vi "get.vi"(8 "variableArray":string[][](array[string]), 10 "variables":string[](array[string])=["intout", "stringout", "time"], 11 "Experience ID":string="Test") -> (0 "error out":errorcluster={"status"=TRUE, "code"=1, "source"="Entry not found"}, 2 "values":string[](array[string])=["0"], 3 "names":string[](array[string])=["intout"], 5 "values 2":string[](array[string])=["0"], 7 "names 2":string[](array[string])=["intout"])   [LabVIEW 2020]
panel:
  # "Get"
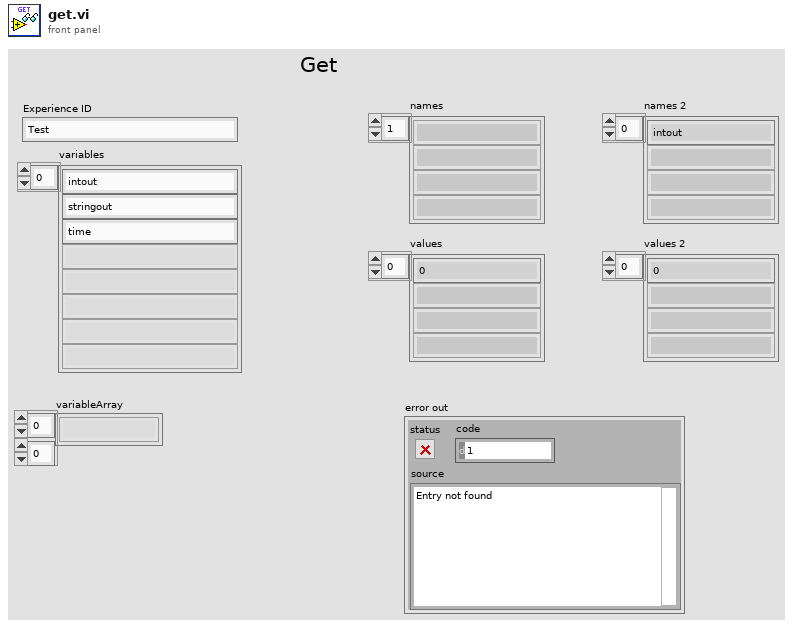
[diagram p1: front panel]
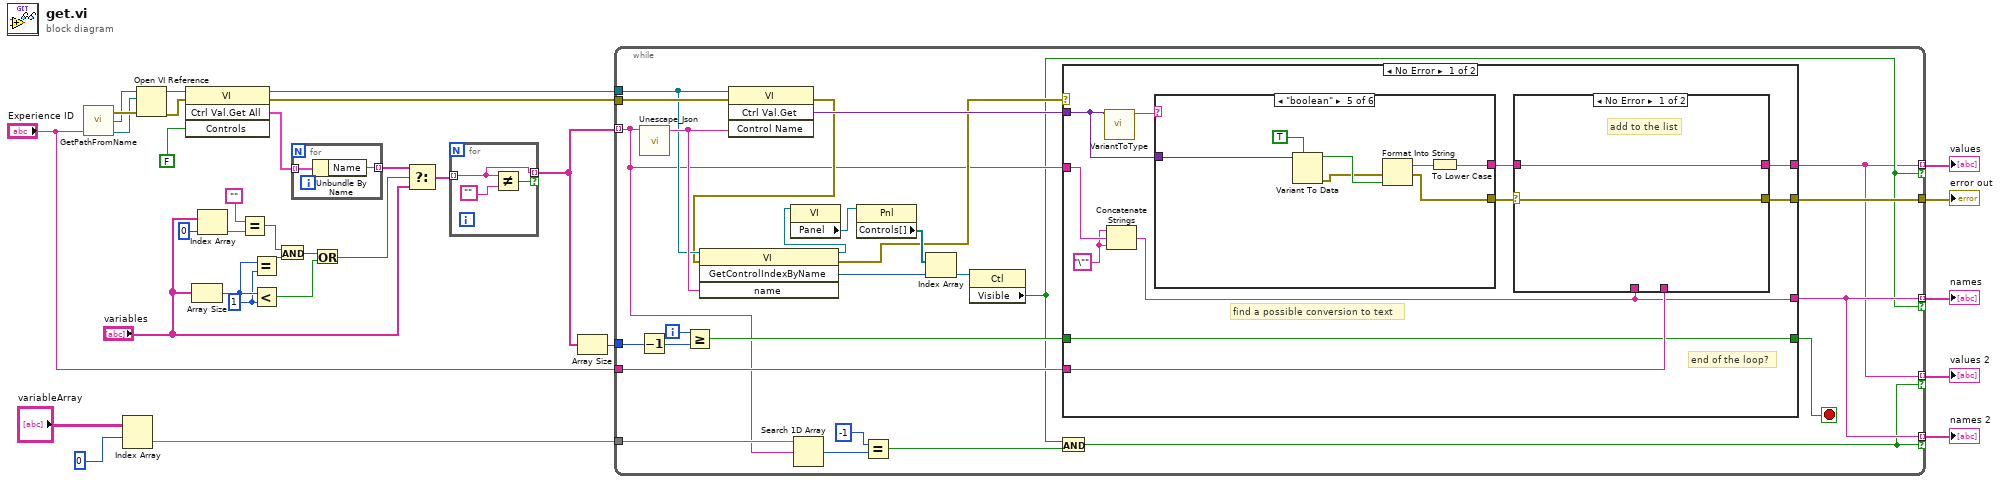
[diagram p0: block diagram]
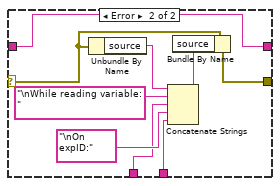
[diagram p2: hidden frame]
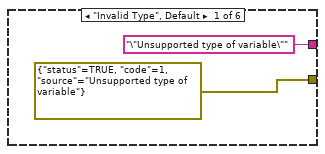
[diagram p3: hidden frame]
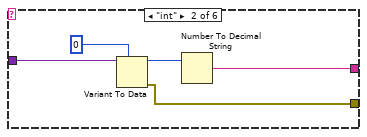
[diagram p4: hidden frame]
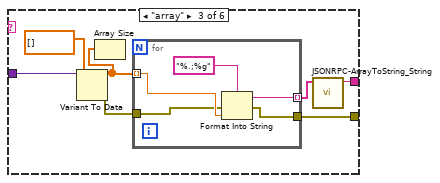
[diagram p5: hidden frame]
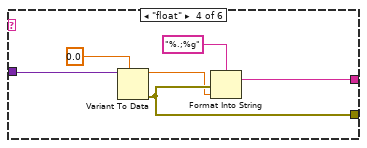
[diagram p6: hidden frame]
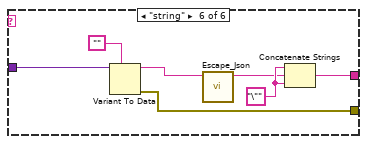
[diagram p7: hidden frame]
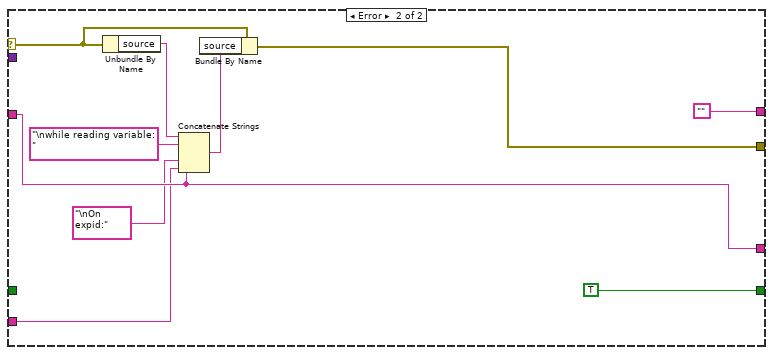
[diagram p8: hidden frame]
diagram:
  w22 = 1 ("y")
  n1 = call "GetPathFromName.vi"("Experience ID"="Experience ID") -> ("VI_Path"=w2:path, "application reference"=w1:refnum<vi>, "Error out"=w3:errorcluster)  [unwired: 2 in]
  n2 = Index Array(array="variableArray", index (row)=0) -> (element=w7:string[])  [unwired: 1 in]
  n3 = Open VI Reference(application reference (local)=w1, vi path=w2, error in (no error)=w3) -> (vi reference=w29:refnum<vi>, error out=w19:errorcluster)  [unwired: 3 out]
  n4 = invoke class="VI" method="Ctrl Val.Get All"(reference=w29, error in=w19, "Controls"=FALSE) -> (reference out=w28:refnum<vi>, error out=w18:errorcluster, "Get All Control Values Variant"=w26:cluster{"Name":string, "Variant Data":variant}[])  [unwired: 1 in, 1 out]
  n5 = Array Size(array="variables") -> (size(s)=w23:i32)
  n6 = Index Array(array="variables", index=0) -> (element=w13:string)
  n7 = Equal?(x="", y=w13) -> (x = y?=w16:bool)
  n8 = Equal?(x=w23, y=w22) -> (x = y?=w20:bool)
  n9 = Less?(x=w23, y=w22) -> (x < y?=w24:bool)
  n10 = And(x=w16, y=w20) -> (x .and. y?=w21:bool)
  n11 = for {
    tunnel: w26 -> [w35] mode=indexing
    tunnel: [w34] -> w25 mode=indexing
    n12 = Unbundle By Name(w35) -> ("Name"=w34:string)
  }
  n13 = Or(x=w21, y=w24) -> (x .or. y?=w12:bool)
  n14 = Select(t=w25, s=w12, f="variables") -> (s? t:f=w11:string[])
  n15 = for {
    tunnel: w11 -> [w37] mode=indexing
    tunnel: [w37] -> w10 mode=indexing if=w36
    n16 = Not Equal?(x=w37, y="") -> (x != y?=w36:bool)
  }
  n17 = Array Size(array=w10) -> (size(s)=w33:i32)
  n18 = while {
    tunnel: w10 -> [w46] mode=indexing
    tunnel: w28 -> [w53]
    tunnel: w33 -> [w60]
    tunnel: w18 -> [w65]
    tunnel: [w62] -> w30
    tunnel: [w40] -> w32 mode=indexing if=w42
    tunnel: [w43] -> w31 mode=indexing if=w42
    tunnel: "Experience ID" -> [w61]
    tunnel: w7 -> [w47]
    tunnel: [w43] -> w6 mode=indexing if=w39
    tunnel: [w40] -> w5 mode=indexing if=w39
    i -> [w48]
    stop <- w63 stop-if-true
    n19 = Decrement(x=w60) -> (x-1=w58:i32)
    n20 = call "Unescape_Json.vi"("Json_String"=w46) -> ("String"=w54:string)  [unwired: 9 in]
    n21 = Greater Or Equal?(x=w48, y=w58) -> (x >= y?=w59:bool)
    n22 = invoke class="VI" method="Ctrl Val.Get"(reference=w53, error in=w65, "Control Name"=w54) -> (error out=w50:errorcluster, "Get Control Value Variant"=w64:variant)  [unwired: 1 in, 2 out]
    n23 = invoke class="VI" method="GetControlIndexByName"(reference=w53, error in=w50, "name"=w54) -> (reference out=w51:refnum<vi>, error out=w49:errorcluster, "GetControlIndexByName"=w57:i32)  [unwired: 1 in, 1 out]
    n24 = property class="VI"(reference=w51) -> ("Panel"=w52:refnum<vi>)  [unwired: 1 in, 2 out]
    n25 = Search 1D Array(1D array=w47, element=w46) -> (index of element=w45:i32)  [unwired: 1 in]
    n26 = property class="Pnl"(reference=w52) -> ("Controls[]"=w56:refnum<vi>[])  [unwired: 1 in, 2 out]
    n27 = Equal?(x=-1, y=w45) -> (x = y?=w41:bool)
    n28 = Index Array(array=w56, index=w57) -> (element=w55:refnum<vi>)
    n29 = property class="Ctl"(reference=w55) -> ("Visible"=w42:bool)  [unwired: 1 in, 2 out]
    n30 = And(x=w42, y=w41) -> (x .and. y?=w39:bool)
    n31 = case shown="No Error" w49 {
      selector: w49 -> [_ w135]
      tunnel: w64 -> [w68 _]
      tunnel: w59 -> [w66 _]
      tunnel: [w66 TRUE] -> w63
      tunnel: w46 -> [w70 w130]
      tunnel: [w75 w131] -> w62
      tunnel: [w73 ""] -> w40
      tunnel: [w71 w130] -> w43
      tunnel: w61 -> [w72 w127]
      frame No Error {
        w69 = "\"" ("string")
        # "end of the loop?"
        # "find a possible conversion to text"
        n32 = call "VariantToType.vi"("Variant"=w68) -> ("type Name"=w67:string)  [unwired: 10 in]
        n33 = Concatenate Strings(w69, w70, w69) -> (w71:string)
        n34 = case shown="\"boolean\"" w67 {
          tunnel: w68 -> [_ w93 w101 w111 w117 w125]
          tunnel: ["\"Unsupported type of variable\"" w91 w96 w107 w113 w122] -> w74
          tunnel: [errorcluster {"status"=TRUE, "code"=1, "source"="Unsupported type of variable"} ("error out") w90 w97 w110 w115 w124] -> w76
          frame "Invalid Type", Default {
          }
          frame "int" {
            n35 = Variant To Data(type=0, Variant=w93) -> (data=w92:i32, error out=w90:errorcluster)  [unwired: 1 in]
            n36 = Number To Decimal String(number=w92) -> (decimal integer string=w91:string)  [unwired: 1 in]
          }
          frame "array" {
            n37 = Variant To Data(type=dbl[] [] ("Array"), Variant=w101) -> (data=w99:dbl[], error out=w98:errorcluster)  [unwired: 1 in]
            n38 = Array Size(array=w99) -> ()  [unwired: 1 out]
            n39 = for {
              tunnel: w99 -> [w105] mode=indexing
              tunnel: w98 -> [w104]
              tunnel: [w103] -> w97
              tunnel: [w102] -> w95 mode=indexing
              n40 = Format Into String(format string="%.;%g", error in=w104, w105) -> (resulting string=w102:string, error out=w103:errorcluster)  [unwired: 1 in]
            }
            n41 = call "JSONRPC-ArrayToString_String.vi"("Array"=w95) -> ("Output"=w96:string)  [unwired: 10 in]
          }
          frame "float" {
            n42 = Variant To Data(type=0.0, Variant=w111) -> (data=w109:dbl, error out=w110:errorcluster)  [unwired: 1 in]
            n43 = Format Into String(format string="%.;%g", error in=w110, w109) -> (resulting string=w107:string)  [unwired: 1 in, 1 out]
          }
          frame "boolean" {
            n44 = Variant To Data(type=TRUE, Variant=w117) -> (data=w119:bool, error out=w118:errorcluster)  [unwired: 1 in]
            n45 = Format Into String(error in=w118, w119) -> (resulting string=w114:string, error out=w115:errorcluster)  [unwired: 2 in]
            n46 = To Lower Case(string=w114) -> (all lower case string=w113:string)
          }
          frame "string" {
            w123 = "\"" ("string")
            n47 = Variant To Data(type="", Variant=w125) -> (data=w120:string, error out=w124:errorcluster)  [unwired: 1 in]
            n48 = call "Escape_Json.vi"("String"=w120) -> ("Json_string"=w121:string)  [unwired: 9 in]
            n49 = Concatenate Strings(w123, w121, w123) -> (w122:string)
          }
        }
        n50 = case shown="No Error" w76 {
          selector: w76 -> [w78 w86]
          tunnel: [w78 w87] -> w75
          tunnel: [w77 w79] -> w73
          tunnel: w74 -> [w77 w79]
          tunnel: w71 -> [_ w81]
          tunnel: w72 -> [_ w80]
          frame No Error {
            # "add to the list"
          }
          frame Error {
            n51 = Unbundle By Name(w86) -> ("source"=w85:string)
            n52 = Concatenate Strings(w85, "\nWhile reading variable: " ("string"), w81, "\nOn expID:" ("string"), w80) -> (w83:string)
            n53 = Bundle By Name(cluster=w86, "source"=w83) -> (w87:errorcluster)
          }
        }
      }
      frame Error {
        n54 = Unbundle By Name(w135) -> ("source"=w134:string)
        n55 = Concatenate Strings(w134, "\nwhile reading variable: " ("string"), w130, "\nOn expid:", w127) -> (w132:string)
        n56 = Bundle By Name(cluster=w135, "source"=w132) -> (w131:errorcluster)
      }
    }
  }
  "error out" <- w30
  "names" <- w31
  "values" <- w32
  "names 2" <- w6
  "values 2" <- w5
